vi "NML_ASRL_Scan.vi"() -> ()   [LabVIEW 2025]
doc: "Scans all primary addresses on the GPIB bus and reports status of devices found there.\nScott Hannahs, F. Bitter National Magnet Lab, April 1993\nAuthor: Scott Hannahs <sth@magnet.fsu.edu>\n\nThis software is licensed for use under the “MIT License\"\nCopyright (c) 2025 Scott Hannahs, sth@sth@magnet.sthnet.net\n\nPermission is hereby granted, free of charge, to any person obtaining a copy of this software and associated documentation files (the \"Software\"), to deal in the Software without restriction, including without limitation the rights to use, copy, modify, merge, publish, distribute, sublicense, and/or sell copies of the Software, and to permit persons to whom the Software is furnished to do so, subject to the following conditions: The above copyright notice and this permission notice shall be included in all copies or substantial portions of the Software.\n\nTHE SOFTWARE IS PROVIDED \"AS IS\", WITHOUT WARRANTY OF ANY KIND, EXPRESS OR IMPLIED, INCLUDING BUT NOT LIMITED TO THE WARRANTIES OF MERCHANTABILITY, FITNESS FOR A PARTICULAR PURPOSE AND NONINFRINGEMENT. IN NO EVENT SHALL THE AUTHORS OR COPYRIGHT HOLDERS BE LIABLE FOR ANY CLAIM, DAMAGES OR OTHER LIABILITY, WHETHER IN AN ACTION OF CONTRACT, TORT OR OTHERWISE, ARISING FROM, OUT OF OR IN CONNECTION WITH THE SOFTWARE OR THE USE OR OTHER DEALINGS IN THE SOFTWARE."
panel:
  in  "Run":bool
  out "Serial Port List:":T1(array[cluster])
  out "error out":errorcluster
  # "USE FOR BLM ONLY"
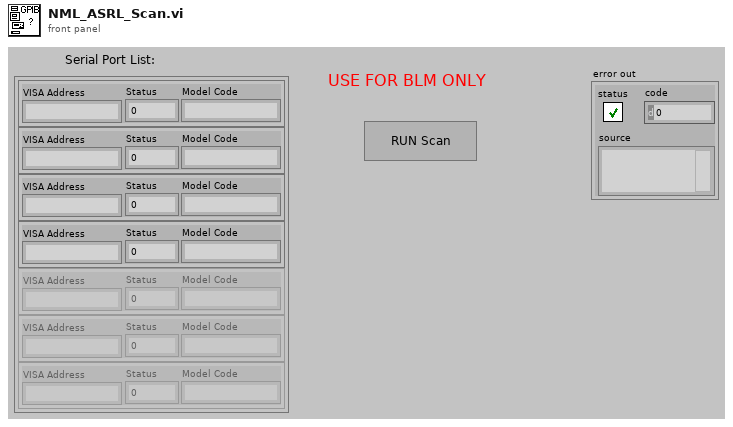
[diagram p1: front panel]
types:
  T1 = cluster{"VISA Address":string, "Status":u16, "Model Code":string}[]
  T2 = cluster{"VISA Address":string, "Status":u16, "Manufacturer":string}[]
  T3 = cluster{refnum<visa-resource-name>, i32, "String Returned":string}
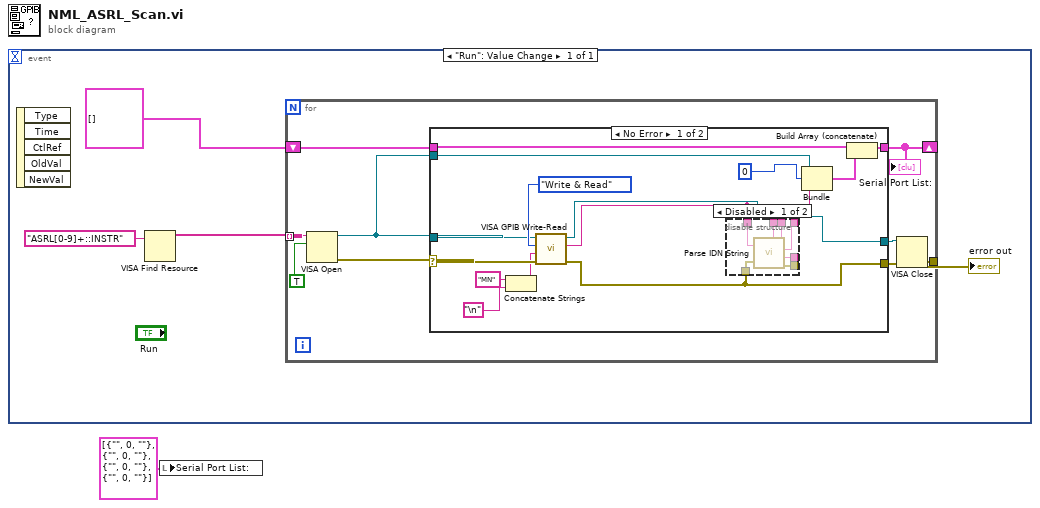
[diagram p0: block diagram]
diagram:
  n1 = event shown="[0] \"Run\": Value Change" {
    selector: _ -> [_]
    dyn-events: _ -> [_]
    timeout: _ -> [_]
    event "Run": Value Change {
      n2 = event-data() -> ()  [unwired: 1 in, 5 out]
      n3 = VISA Find Resource(11:"ASRL[0-9]+::INSTR" ("expression (\"?*\")")) -> (3:w3:string[])  [unwired: 2 in, 2 out]
      n4 = for {
        tunnel: w3 -> [w9] mode=indexing
        tunnel: [w13] -> w5
        shift-right: [w10] -> _
        shift-left: T2 [] ("Instrument List") -> [w11]
        n5 = VISA Open(duplicate session (F)=TRUE, VISA resource name=w9) -> (VISA resource name=w6:refnum<visa-resource-name>, error out=w7:errorcluster)  [unwired: 3 in]
        n6 = case shown="No Error" w7 {
          selector: w7 -> [w26 w37]
          tunnel: [w19 w37] -> w14
          tunnel: w6 -> [w27 w38]
          tunnel: [w20 w38] -> w12
          tunnel: w11 -> [w24 w36]
          tunnel: [w25 w36] -> w10
          tunnel: w6 -> [w23 _]
          frame No Error {
            n7 = Concatenate Strings("MN" ("write buffer (\"\")"), "\n") -> (w16:string)
            n8 = call "VISA GPIB Write-Read.vi"("error in (no error)"=w26, "Command"=w16, "Action"=enum16{"Write", "Read", "Write & Read"}."Write & Read", "VISA resource name"=w27) -> ("error out"=w19:errorcluster, "String Returned"=w18:string, "dup VISA Session"=w20:refnum<visa-resource-name>)  [unwired: 4 in, 1 out]
            n9 = disable-structure shown="Disabled" {
              disable-tunnel: [w35 _] -> _
              disable-tunnel: [w34 _] -> _
              disable-tunnel: [w33 _] -> _
              disable-tunnel: [w32 _] -> _
              disable-tunnel: [w31 _] -> _
              disable-tunnel: w18 -> [w30 _]
              disable-tunnel: w19 -> [w29 _]
              frame Disabled {
                n10 = call "Parse IDN String.vi"("error in (no error)"=w29, "IDN String"=w30) -> ("error out"=w32:errorcluster, "Info"=w33:string, "Model"=w34:string, "Manufacturer"=w35:string, "Revision"=w31:string)
              }
              frame Enabled {
              }
            }
            n11 = Bundle(w23, 0, "String Returned"=w18) -> (w17:T3)  [unwired: 1 in]
            n12 = Build Array (concatenate)(w24, w17) -> (w25:T2)
          }
          frame Error {
          }
        }
        "Serial Port List:" <- w10
        n13 = VISA Close(VISA resource name=w12, error in (no error)=w14) -> (error out=w13:errorcluster)
      }
      "error out" <- w5
    }
  }
  n14 = local write "Serial Port List:"(T1 [{"VISA Address"="", "Status"=0, "Model Code"=""}, {"VISA Address"="", "Status"=0, "Model Code"=""}, {"VISA Address"="", "Status"=0, "Model Code"=""}, {"VISA Address"="", "Status"=0, "Model Code"=""}] ("Serial Port List:")) -> ()
